vi "yakup_demiryurek.vi"() -> ()   [LabVIEW 2020]
panel:
  out "?":string
  out "Asal mı?":bool
  in  "Sayı Giriniz":i64
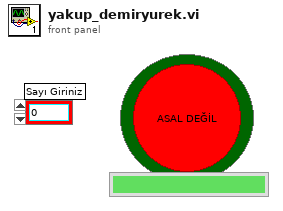
[diagram p1: front panel]
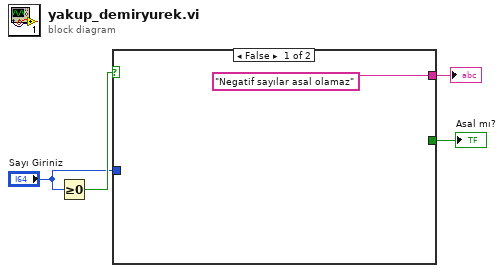
[diagram p0: block diagram]
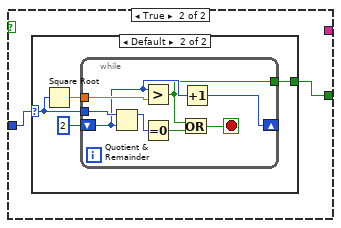
[diagram p2: hidden frame]
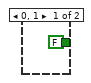
[diagram p3: hidden frame]
diagram:
  n1 = Greater Or Equal To 0?(x="Sayı Giriniz") -> (x >= 0?=w3:bool)
  n2 = case shown="False" w3 {
    tunnel: [_ w7] -> w4
    tunnel: "Sayı Giriniz" -> [_ w6]
    tunnel: ["Negatif sayılar asal olamaz" _] -> w1
    frame False {
    }
    frame True {
      n3 = case shown="Default" w6 {
        selector: w6 -> [_ w10]
        tunnel: [FALSE w9] -> w7
        frame 0, 1 {
        }
        frame Default {
          n4 = Square Root(x=w10) -> (sqrt(x)=w11:dbl)
          n5 = while {
            shift-right: [w19] -> _
            shift-left: 2 -> [w14]
            tunnel: w10 -> [w18]
            tunnel: w11 -> [w15]
            tunnel: [w13] -> w9
            stop <- w16 stop-if-true
            n6 = Quotient & Remainder(x=w18, y=w14) -> (x-y*floor(x/y)=w20:i64)  [unwired: 1 out]
            n7 = Greater?(x=w14, y=w15) -> (0:w13:bool)
            n8 = Equal To 0?(x=w20) -> (x = 0?=w17:bool)
            n9 = Or(x=w13, y=w17) -> (x .or. y?=w16:bool)
            n10 = Increment(x=w14) -> (x+1=w19:i32)
          }
        }
      }
    }
  }
  "Asal mı?" <- w4
  "?" <- w1
